vi "GlobalControlVariables.vi"() -> ()   [LabVIEW 2016]
panel:
  out "Recv Data":string
  out "Recv Enable":bool
  out "Global Error Message":string
  out "TPC Semaphore":string
  out "Send Data":string
  out "Send Enable":bool
  out "Quit":bool
  in  "TCP error":errorcluster
  out "Default Port":u16
  in  "TCP Refnum":refnum<k5>
  out "Connected?":bool
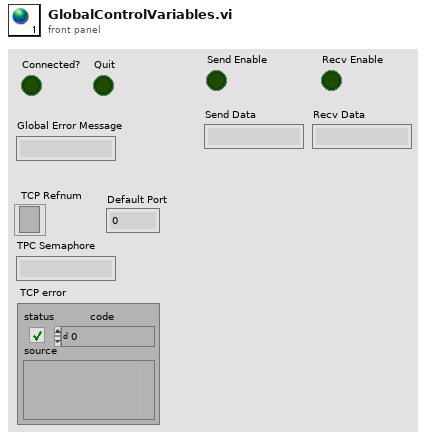
[diagram p1: front panel]
diagram:
